vi "Start Transmit Inline.vi"(8 "error in (no error)":errorcluster, 11 "Plugin in":refnum<class "Plugin.lvclass">) -> (0 "error out":errorcluster, 3 "Plugin out":refnum<class "Plugin.lvclass">)   [LabVIEW 2017, in "Data Sharing Framework Core.lvlib" / "Data Sharing Framework Engine.lvlib" / "Plugin.lvclass"]
uses:
  Plugin.lvclass
  Plugin.lvclass/Plugin.ctl
  Internal/Interfaces/Transceiver Interface/Command.ctl
  Transfer Group/Transfer Group.lvclass/Transfer Group.ctl
  Internal/Timing/Engine Timing.lvclass/Engine Timing.ctl
  Internal/Timing/Increment Iteration Count.vi
  Internal/Interfaces/Transceiver Interface/Transceiver Interface.lvclass
  Transfer Group/Transfer Group.lvclass
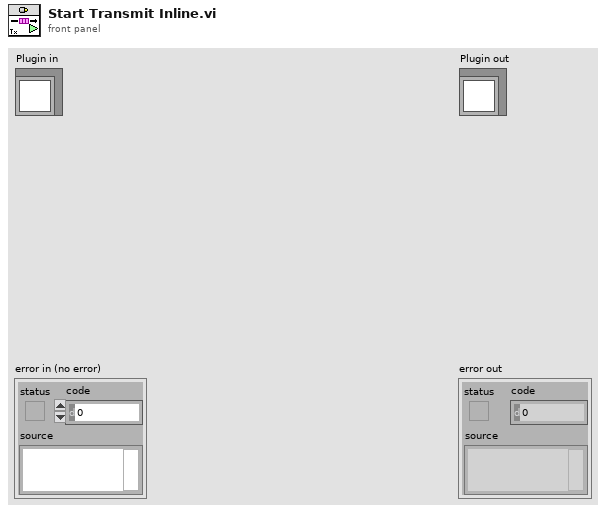
[diagram p1: front panel]
types:
  T1 = typedef "Data Sharing Framework Core.lvlib/Data Sharing Framework Engine.lvlib/Transceiver Interface.lvclass/Command.ctl" = enum8{"Set Base Pointer", "Receive", "Transmit", "Shutdown"}
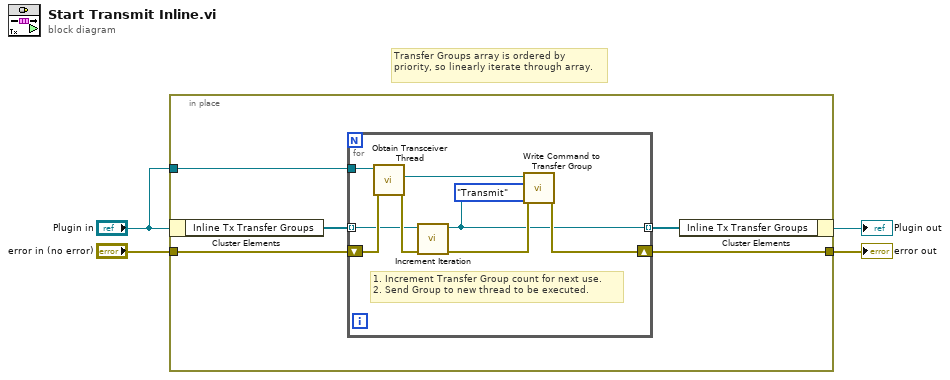
[diagram p0: block diagram]
diagram:
  # "Transfer Groups array is ordered by priority, so linearly iterate through array."
  n1 = in-place {
    in-place-border: "error in (no error)" -> [w9]
    in-place-border: [w8] -> w3
    in-place-border: "Plugin in" -> [w5]
    n2 = in-place-cluster #1("Plugin in") -> ("Inline Tx Transfer Groups"=w7:refnum<class "Transfer Group.lvclass">[])
    n3 = for {
      tunnel: w7 -> [w14] mode=indexing
      shift-right: [w11] -> w8
      shift-left: w9 -> [w16]
      tunnel: [w10] -> w6 mode=indexing
      tunnel: w5 -> [w17]
      # "1. Increment Transfer Group count for next use.\n2. Send Group to new thread to be executed."
      n4 = call "Obtain Transceiver Thread.vi"("error in (no error)"=w16, "Plugin in"=w17) -> ("error out"=w15:errorcluster, "Transceiver Thread"=w18:refnum<class "Transceiver Interface.lvclass">)  [unwired: 7 in, 1 out]
      n5 = call "Increment Iteration.vi"("error in (no error)"=w15, "Transfer Group in"=w14) -> ("error out"=w12:errorcluster, "Transfer Group out"=w10:refnum<class "Transfer Group.lvclass">)  [unwired: 8 in]
      n6 = call "Write Command to Transfer Group.vi"("error in (no error)"=w12, "Command"=Command."Transmit", "Transfer Group"=w10, "Transceiver Interface in"=w18) -> ("error out"=w11:errorcluster)  [unwired: 6 in, 1 out]
    }
    n7 = in-place-cluster #1("Inline Tx Transfer Groups"=w6) -> (→"Plugin out":refnum<class "Plugin.lvclass">)
  }
  "error out" <- w3
